vi "MTM2_getEvent_temperatureOffset.vi"(8 "error in (no error)":errorcluster, 11 "logevent_temperatureOffset_Ctl":T1={"private_rcvStamp"=0.0, "ring[12]"=[0.0, 0.0, 0.0, 0.0, 0.0, 0.0, 0.0, 0.0, 0.0, 0.0, 0.0, 0.0], "intake[2]"=[0.0, 0.0], "exhaust[2]"=[0.0, 0.0], "priority"=0}) -> (0 "error out":errorcluster, 2 "function return":i32, 3 "logevent_temperatureOffset_Ctl out":T1)   [LabVIEW 2018, in "SALLV_MTM2.lvlib"]
doc: "int MTM2_shm_getEvent_temperatureOffsetLV(MTM2_logevent_temperatureOffsetLV *logevent_temperatureOffset_Ctl );"
uses:
  DataTypes/logevent_temperatureOffset.ctl
  SALLV_MTM2.lvlib
  SALLV_MTM2.so
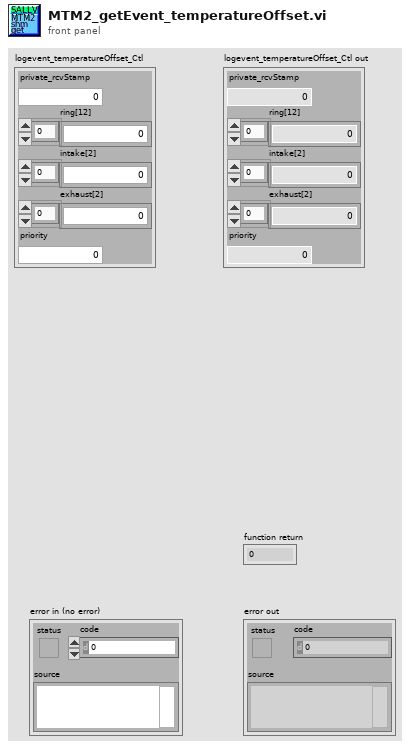
[diagram p1: front panel]
types:
  T1 = typedef "SALLV_MTM2.lvlib/logevent_temperatureOffset.ctl" = cluster{"private_rcvStamp":dbl, "ring[12]":dbl[], "intake[2]":dbl[], "exhaust[2]":dbl[], "priority":i32}
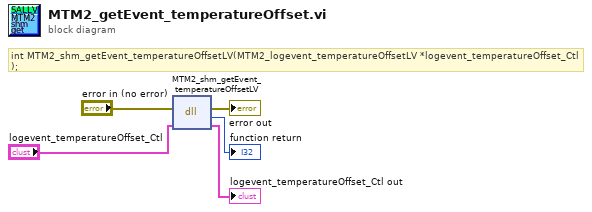
[diagram p0: block diagram]
diagram:
  # "int MTM2_shm_getEvent_temperatureOffsetLV(MTM2_logevent_temperatureOffsetLV *logevent_temperatureOffset_Ctl );"
  n1 = dll-call lib="home/ttsai/Documents/salLabviewApi/SALLV_MTM2/SALLV_MTM2.*" fn="MTM2_shm_getEvent_temperatureOffsetLV"(error in="error in (no error)", "logevent_temperatureOffset_Ctl"="logevent_temperatureOffset_Ctl") -> (error out=→"error out":errorcluster, →"function return":i32, "logevent_temperatureOffset_Ctl"=→"logevent_temperatureOffset_Ctl out":T1)  [unwired: 2 in, 1 out]
